vi "Configure Serial Bus (CXPI - Trigger).vi"(0 "VISA resource name":refnum<visa-resource-name>, 1 "Enable ID Filter (F: Disable)":bool, 5 "Serial Bus Name (1: Serial Bus 1)":i32(ring)=1 items=["Serial Bus 1"=1, "Serial Bus 2"=2], 7 "Trigger Mode (0: Start of Frame)":i32(ring) items=["Start of Frame", "End of Frame", "PTYPE", "Frame ID", "Frame Data", "Long Frame Data", "CRC Field Error", "Parity Error", "Inter-Byte Space Error", "Inter-Frame Space Error", "Frame Error", "Data Length Error", "Sample Error", "All Error", "Sleep Frame", "Wake Up Pulse"], 9 "Frame ID (XXXXXXX)":string="XXXXXXX", 11 "error in (no error)":errorcluster, 12 "Enable PTYPE Trigger (F: Disable)":bool) -> (4 "VISA resource name out":refnum<visa-resource-name>, 15 "error out":errorcluster)   [LabVIEW 2017, in "Agilent 2000 3000 X-Series.lvlib"]
doc: "Configures the trigger setting of CXPI bus.\n\n<b>Note:</b>\nThis VI is only applicable for 3000T, 4000, 6000 X-Series."
uses:
  Agilent 2000 3000 X-Series.lvlib
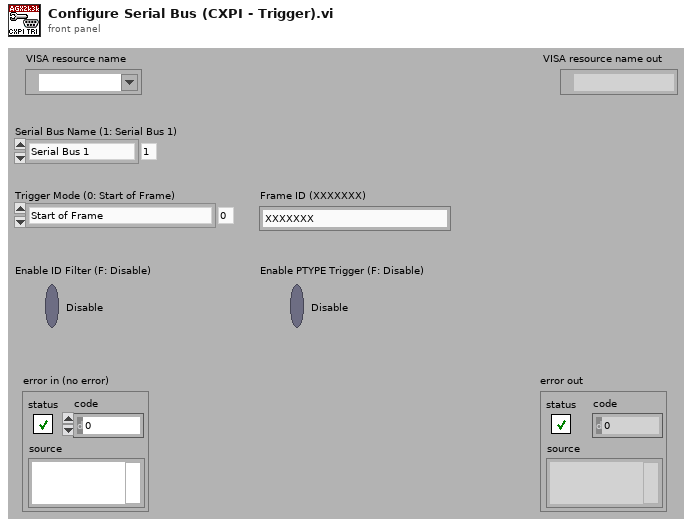
[diagram p1: front panel]
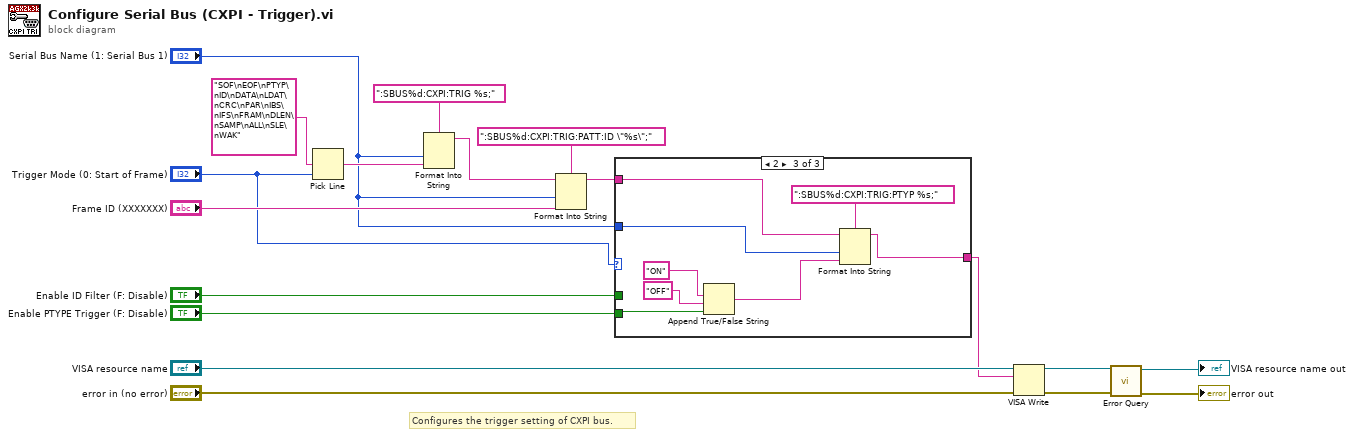
[diagram p0: block diagram]
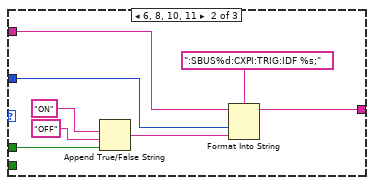
[diagram p3: hidden frame]
diagram:
  # "Configures the trigger setting of CXPI bus."
  n1 = Pick Line(multi-line string="SOF\nEOF\nPTYP\nID\nDATA\nLDAT\nCRC\nPAR\nIBS\nIFS\nFRAM\nDLEN\nSAMP\nALL\nSLE\nWAK", line index="Trigger Mode (0: Start of Frame)") -> (output string=w16:string)  [unwired: 1 in]
  n2 = Format Into String(format string=":SBUS%d:CXPI:TRIG %s;", "Serial Bus Name (1: Serial Bus 1)", w16) -> (resulting string=w5:string)  [unwired: 2 in, 1 out]
  n3 = Format Into String(format string=":SBUS%d:CXPI:TRIG:PATT:ID \"%s\";", initial string=w5, "Serial Bus Name (1: Serial Bus 1)", "Frame ID (XXXXXXX)") -> (resulting string=w4:string)  [unwired: 1 in, 1 out]
  n4 = case shown="2" "Trigger Mode (0: Start of Frame)" {
    tunnel: "Enable ID Filter (F: Disable)" -> [_ w23 _]
    tunnel: "Enable PTYPE Trigger (F: Disable)" -> [_ _ w31]
    tunnel: [w19 w22 w28] -> w1
    tunnel: w4 -> [w19 w21 w30]
    tunnel: "Serial Bus Name (1: Serial Bus 1)" -> [_ w20 w29]
    frame 0, Default {
    }
    frame 6, 8, 10, 11 {
      n5 = Append True/False String(1:w23, 2:"OFF", 3:"ON") -> (0:w27:string)  [unwired: 1 in]
      n6 = Format Into String(format string=":SBUS%d:CXPI:TRIG:IDF %s;", initial string=w21, w20, w27) -> (resulting string=w22:string)  [unwired: 1 in, 1 out]
    }
    frame 2 {
      n7 = Append True/False String(1:w31, 2:"OFF", 3:"ON") -> (0:w35:string)  [unwired: 1 in]
      n8 = Format Into String(format string=":SBUS%d:CXPI:TRIG:PTYP %s;", initial string=w30, w29, w35) -> (resulting string=w28:string)  [unwired: 1 in, 1 out]
    }
  }
  n9 = VISA Write(VISA resource name="VISA resource name", write buffer=w1, error in (no error)="error in (no error)") -> (VISA resource name out=w9:refnum<visa-resource-name>, error out=w8:errorcluster)  [unwired: 1 out]
  n10 = call "Error Query.vi"("error in (no error)"=w8, "VISA resource name"=w9) -> ("error out"=→"error out":errorcluster, "VISA resource name out"=→"VISA resource name out":refnum<visa-resource-name>)  [unwired: 6 in, 2 out]
